vi "detrend.vi"(9 "Detrend mode":T1=enum."Linear", 11 "Input":dbl[](array[numeric])) -> (1 "intercept":dbl, 2 "slope":dbl, 3 "Output":dbl[](array[numeric]))   [LabVIEW 2014]
uses:
  detrend_mode.ctl
  <vilib>/Analysis/6fits.llb/Curve Fitting Criteria.ctl
  <vilib>/Analysis/NI_AALPro.lvlib
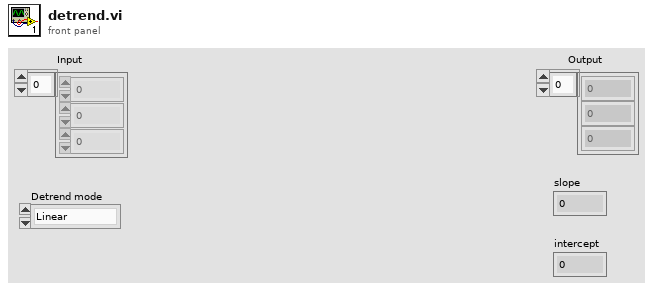
[diagram p1: front panel]
types:
  T1 = typedef "detrend_mode.ctl" = enum16{"Zero mean", "Linear", "Robust linear"}
  T2 = typedef "NI_AALPro.lvlib/Curve Fitting Criteria.ctl" = u16
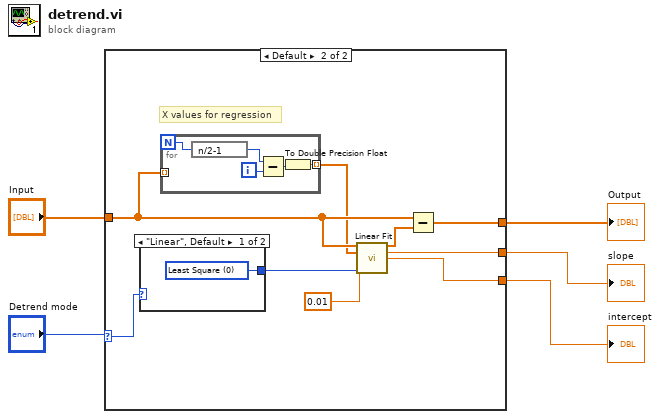
[diagram p0: block diagram]
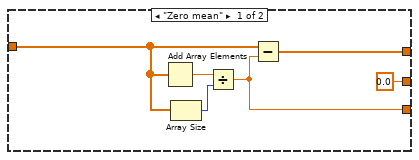
[diagram p2: hidden frame]
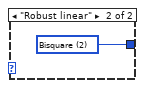
[diagram p3: hidden frame]
diagram:
  n1 = case shown="Default" "Detrend mode" {
    selector: "Detrend mode" -> [_ w12]
    tunnel: "Input" -> [w9 w20]
    tunnel: [w8 w19] -> w4
    tunnel: [w6 w14] -> w3
    tunnel: [0.0 ("slope") w13] -> w2
    frame "Zero mean" {
      n2 = Add Array Elements(numeric array=w9) -> (sum=w10:dbl)
      n3 = Array Size(array=w9) -> (size(s)=w11:i32)
      n4 = Divide(x=w10, y=w11) -> (x/y=w6:dbl)
      n5 = Subtract(x=w9, y=w6) -> (x-y=w8:dbl[])
    }
    frame Default {
      # "X values for regression"
      n6 = case shown="\"Linear\", Default" w12 {
        tunnel: [w21 w22] -> w17
        frame "Linear", Default {
          w21 = T2 0 items=["Least Square", "Least Absolute Residual", "Bisquare"] ("method")
        }
        frame "Robust linear" {
          w22 = T2 2 items=["Least Square", "Least Absolute Residual", "Bisquare"] ("method")
        }
      }
      n7 = for {
        N -> [w26]
        tunnel: w20 -> [_] mode=indexing
        tunnel: [w27] -> w18 mode=indexing
        i -> [w25]
        n8 = expression code="n/2-1"(w26) -> (w23:i32)
        n9 = Subtract(x=w23, y=w25) -> (x-y=w24:i32)
        n10 = To Double Precision Float(number=w24) -> (double precision float=w27:dbl)
      }
      n11 = call <vilib>:"Linear Fit.vi"("Y"=w20, "X"=w18, "tolerance"=0.01, "method"=w17) -> ("Best Linear Fit"=w15:dbl[], "slope"=w13:dbl, "intercept"=w14:dbl)  [unwired: 7 in, 2 out]
      n12 = Subtract(x=w20, y=w15) -> (x-y=w19:dbl[])
    }
  }
  "Output" <- w4
  "intercept" <- w3
  "slope" <- w2
